vi "FPGA-6682PPS.vi"() -> ()   [LabVIEW 2016]
uses:
  <vilib>/userdefined/High Color/nirio_resource_hc.ctl
  <instrlib>/niSync/niSync.llb/niSync Initialize (IVI).vi
  <instrlib>/niSync/niSync.llb/niSync Set Time Reference (1588 Ordinary Clock).vi
  <vilib>/FPGAPlugInAG/PXIe-6592R/niLvFpga_Open_PXIe-6592R.vi
  <vilib>/rvi/interface/common/dynamic/niFpgaDynamicAddResources.vi
  <vilib>/FPGAPlugInAG/Dynamic/niLvFpga_Reset_Dynamic.vi
  <vilib>/FPGAPlugInAG/Dynamic/niLvFpga_Run_Dynamic.vi
  <vilib>/FPGAPlugInAG/Dynamic/niLvFpga_Close_Dynamic.vi
  <vilib>/rvi/interface/nirviOpenFPGA/nirviOpenFPGA.xnode
  FPGA Bitfiles/8021ASPXIe_FPGATarget_PPSTimeKeeper_QOpza4nxlo4.lvbitx
  FPGA/PPS TimeKeeper.vi
  <vilib>/rvi/interface/nirviMethod/nirviMethod.xnode
  <vilib>/rvi/interface/nirviCloseFPGA/nirviCloseFPGA.xnode
panel:
  out "FPGA Time":timestamp
  out "6683 Time":timestamp
  in  "sync abs time":bool
  in  "FTE Terminal":tag="/Dev1/PXI_Trig7"
  out "error out":errorcluster
  in  "stop":bool
  in  "Sync Board Name":refnum<k15>="PXI1Slot2"
  in  "FPGA Name":T1
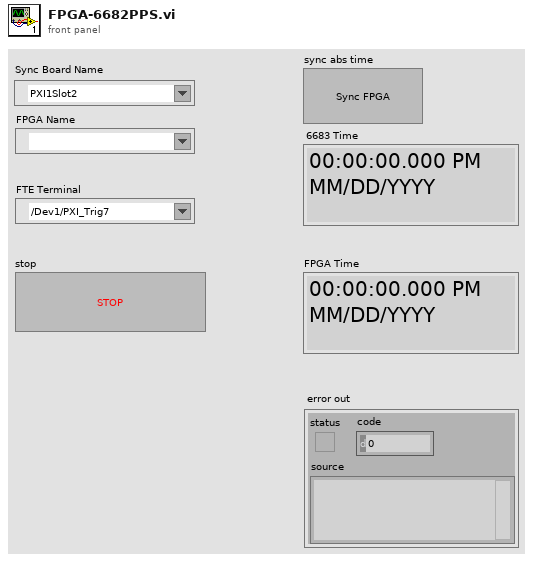
[diagram p1: front panel]
types:
  T1 = typedef "nirio_resource_hc.ctl" = tag
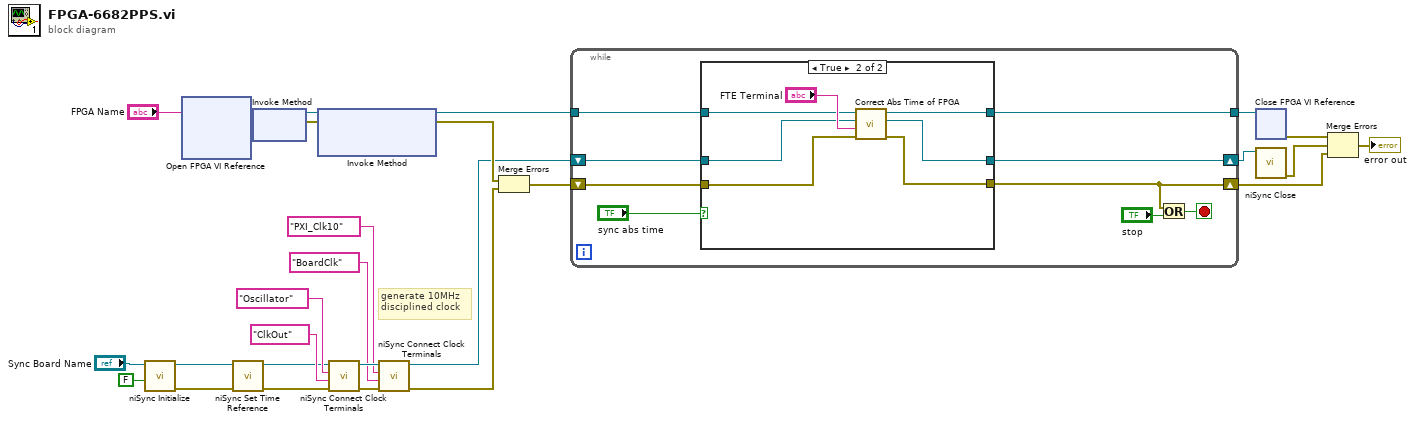
[diagram p0: block diagram]
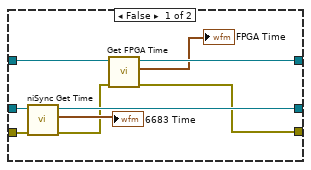
[diagram p2: hidden frame]
diagram:
  # "generate 10MHz \ndisciplined clock"
  n1 = call-poly <instrlib>:"niSync Initialize.vi"("reset device (F)"=FALSE ("reset device (False)"), "resource name"="Sync Board Name") -> ("error out"=w19:errorcluster, "instrument handle out"=w18:refnum<k15>)  [unwired: 8 in]
  n2 = xnode "Open FPGA VI Reference"("resource name"="FPGA Name") -> ("FPGA VI Reference Out"=w9:refnum<k20>, "error out"=w8:errorcluster)  [unwired: 1 in]
  n3 = call-poly <instrlib>:"niSync Set Time Reference.vi"("error in (no error)"=w19, "instrument handle"=w18) -> ("error out"=w16:errorcluster, "instrument handle out"=w17:refnum<k15>)  [unwired: 8 in]
  n4 = xnode "Invoke Method"("FPGA VI Reference In"=w9, "error in"=w8) -> ("FPGA VI Reference Out"=w7:refnum<k20>, "error out"=w6:errorcluster)
  n5 = xnode "Invoke Method"("FPGA VI Reference In"=w7, "error in"=w6) -> ("FPGA VI Reference Out"=w15:refnum<k20>, "error out"=w11:errorcluster)  [unwired: 1 in]
  n6 = call <instrlib>:"niSync Connect Clock Terminals.vi"("error in (no error)"=w16, "destination terminal"="ClkOut", "source terminal"="Oscillator", "instrument handle"=w17) -> ("error out"=w25:errorcluster, "instrument handle out"=w24:refnum<k15>)  [unwired: 6 in]
  n7 = call <instrlib>:"niSync Connect Clock Terminals.vi"("error in (no error)"=w25, "destination terminal"="BoardClk", "source terminal"="PXI_Clk10", "instrument handle"=w24) -> ("error out"=w1:errorcluster, "instrument handle out"=w2:refnum<k15>)  [unwired: 6 in]
  n8 = Merge Errors(w11, w1) -> (w12:errorcluster)
  n9 = while {
    tunnel: w15 -> [w36]
    shift-right: [w30] -> w5
    shift-left: w12 -> [w35]
    shift-right: [w34] -> w13
    shift-left: w2 -> [w37]
    tunnel: [w33] -> w14
    stop <- w31 stop-if-true
    n10 = case shown="True" "sync abs time" {
      tunnel: w37 -> [w46 w49]
      tunnel: w36 -> [w42 w50]
      tunnel: w35 -> [w45 w51]
      tunnel: [w44 w47] -> w34
      tunnel: [w39 w53] -> w30
      tunnel: [w40 w48] -> w33
      frame False {
        n11 = call <instrlib>:"niSync Get Time.vi"("error in (no error)"=w45, "instrument handle"=w46) -> ("error out"=w41:errorcluster, "time"=→"6683 Time":timestamp, "instrument handle out"=w44:refnum<k15>)  [unwired: 5 in]
        n12 = call "Get FPGA Time.vi"("error in"=w41, "Session In"=w42) -> ("error out"=w39:errorcluster, "Time Stamp"=→"FPGA Time":timestamp, "Session Out"=w40:refnum<k20>)  [unwired: 7 in]
      }
      frame True {
        n13 = call "Correct Abs Time of FPGA.vi"("error in"=w51, "FTE Terminal"="FTE Terminal", "IVI Refnum in"=w49, "Session In"=w50) -> ("error out"=w53:errorcluster, "IVI Refnum out"=w47:refnum<k15>, "Session Out"=w48:refnum<k20>)  [unwired: 5 in]
      }
    }
    n14 = Or(x=w30, y="stop") -> (x .or. y?=w31:bool)
  }
  n15 = xnode "Close FPGA VI Reference"("FPGA VI Reference In"=w14) -> ("error out"=w4:errorcluster)  [unwired: 1 in]
  n16 = call <instrlib>:"niSync Close.vi"("instrument handle"=w13) -> ("error out"=w3:errorcluster)  [unwired: 10 in]
  n17 = Merge Errors(w4, w3, w5) -> (→"error out":errorcluster)
